vi "build_array.vi"() -> ()   [LabVIEW 2019]
panel:
  out "Districts":i32[](array[numeric])
  in  "N":dbl
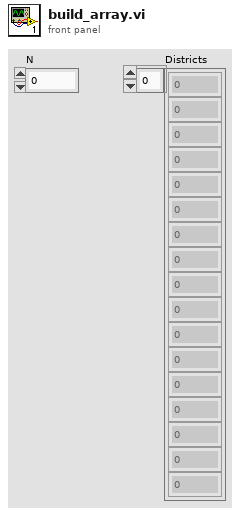
[diagram p1: front panel]
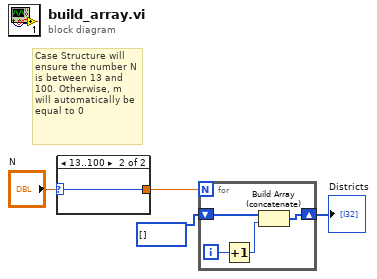
[diagram p0: block diagram]
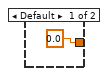
[diagram p2: hidden frame]
diagram:
  # "Case Structure will ensure the number N is between 13 and 100. Otherwise, m will automatically be equal to 0"
  n1 = case shown="13..100" "N" {
    selector: "N" -> [_ w6]
    tunnel: [0.0 w6] -> w2
    frame Default {
    }
    frame 13..100 {
    }
  }
  n2 = for {
    N: w2 -> [_]
    shift-right: [w7] -> w3
    shift-left: i32[] [] -> [w8]
    i -> [w10]
    n3 = Increment(x=w10) -> (x+1=w9:i32)
    n4 = Build Array (concatenate)(w8, w9) -> (w7:i32[])
  }
  "Districts" <- w3
